vi "Write FPGA Interface.vi"(8 "error in (no error)":errorcluster, 10 "FPGA Interface":T1, 11 "FPGA-Bus_Boolean in":refnum<class "FPGA-Bus_I8.lvclass">) -> (0 "error out":errorcluster, 3 "FPGA-Bus_Boolean out":refnum<class "FPGA-Bus_I8.lvclass">)   [LabVIEW 2021, in "FPGA-Bus_I8.lvclass"]
uses:
  FPGA-Bus_I8.lvclass
  Support/FPGA Type.ctl
  FPGA-Bus_I8.lvclass/FPGA-Bus_I8.ctl
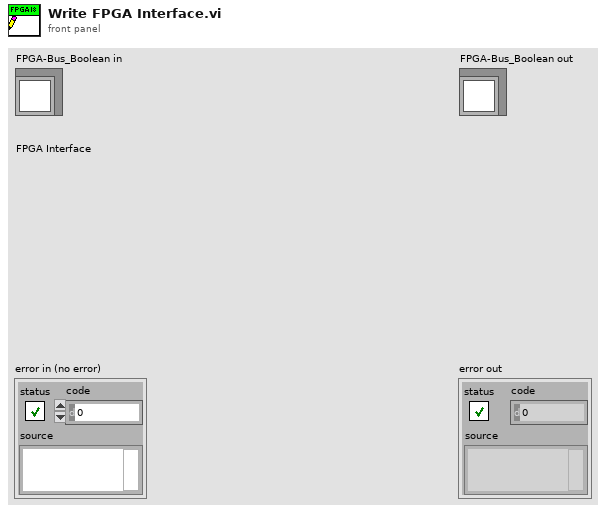
[diagram p1: front panel]
types:
  T1 = typedef "FPGA-Bus_I8.lvclass/FPGA Type.ctl" = refnum<k20>
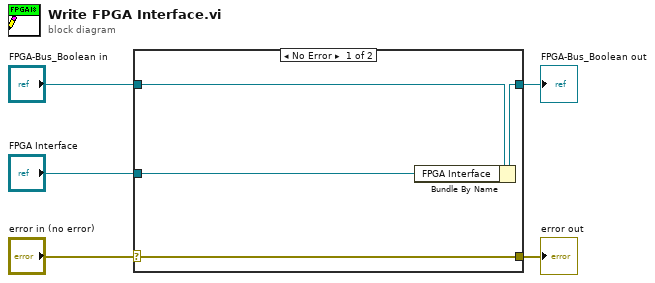
[diagram p0: block diagram]
diagram:
  n1 = case shown="No Error" "error in (no error)" {
    selector: "error in (no error)" -> [w9 w10]
    tunnel: [w9 w10] -> w4
    tunnel: [w7 w11] -> w2
    tunnel: "FPGA-Bus_Boolean in" -> [w8 w11]
    tunnel: "FPGA Interface" -> [w6 _]
    frame No Error {
      n2 = Bundle By Name(cluster=w8, "FPGA Interface"=w6) -> (w7:refnum<class "FPGA-Bus_I8.lvclass">)
    }
    frame Error {
    }
  }
  "error out" <- w4
  "FPGA-Bus_Boolean out" <- w2
